vi "Timer (SubVI).vi"(1 "reset":bool) -> (0 "Is over":bool)   [LabVIEW 2017]
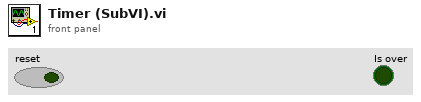
[diagram p1: front panel]
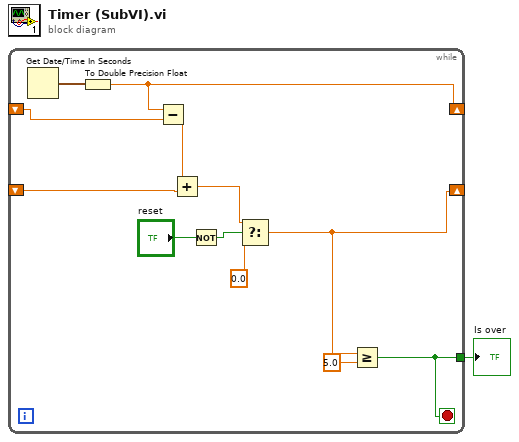
[diagram p0: block diagram]
diagram:
  n1 = while {
    shift-right: [w12] -> _
    shift-left: _ -> [w11]
    shift-right: [w5] -> _
    shift-left: _ -> [w10]
    tunnel: [w4] -> w1
    stop <- w4 stop-if-true
    n2 = Get Date/Time In Seconds() -> (seconds since 1Jan1904=w13:timestamp)
    n3 = To Double Precision Float(number=w13) -> (double precision float=w12:dbl)
    n4 = Subtract(x=w12, y=w11) -> (x-y=w9:dbl)
    n5 = Add(x=w9, y=w10) -> (x+y=w8:dbl)
    n6 = Not(x="reset") -> (.not. x?=w2:bool)
    n7 = Select(t=w8, s=w2, f=0.0) -> (s? t:f=w5:dbl)
    n8 = Greater Or Equal?(x=w5, y=5.0) -> (x >= y?=w4:bool)
  }
  "Is over" <- w1
